vi "出账查询.vi"(9 "结束时间":timestamp format="%<%H:%M\n%y/%m/%d>T", 10 "起始时间":timestamp format="%<%H:%M\n%y/%m/%d>T", 11 "可选条件":bool) -> (1 "查询结果":string[][](table))   [LabVIEW 2010]
panel:
  out "error in (no error)":errorcluster caption="错误输入（无错误）"
  in  "表格控件":string[][](table)
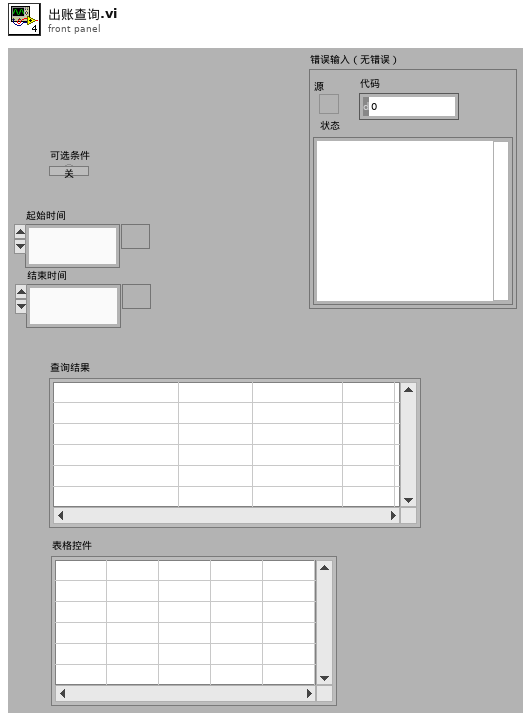
[diagram p1: front panel]
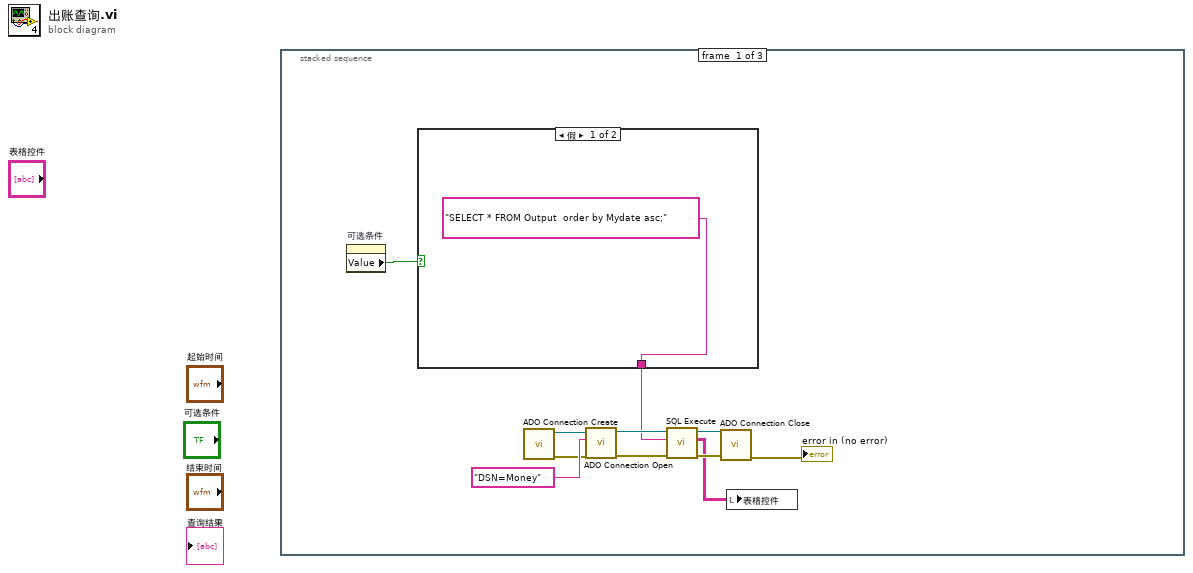
[diagram p0: block diagram]
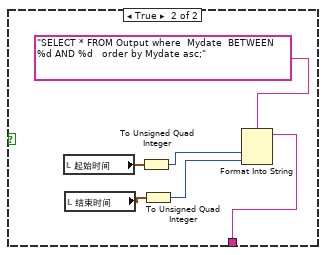
[diagram p2: hidden frame]
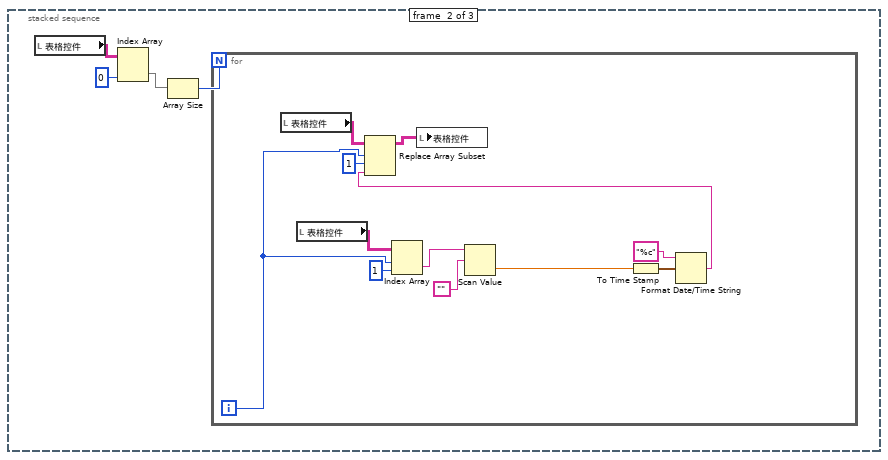
[diagram p3: hidden frame]
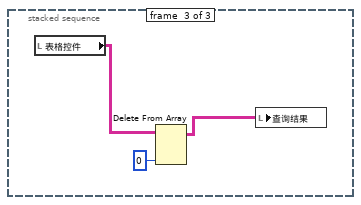
[diagram p4: hidden frame]
diagram:
  n1 = stacked-sequence {
    frame #0 {
      n2 = property on="可选条件" class="Bool (严格)"() -> ("Value"=w3:bool)  [unwired: 2 in, 2 out]
      n3 = case shown="假" w3 {
        tunnel: ["SELECT * FROM Output  order by Mydate asc;" w17] -> w2
        frame False {
        }
        frame True {
          n4 = local read "起始时间"() -> (w16:timestamp)
          n5 = local read "结束时间"() -> (w14:timestamp)
          n6 = To Unsigned Quad Integer(1:w16) -> (0:w15:u64)
          n7 = To Unsigned Quad Integer(1:w14) -> (0:w13:u64)
          n8 = Format Into String(format string="SELECT * FROM Output where  Mydate  BETWEEN %d AND %d   order by Mydate asc;", w15, w13) -> (resulting string=w17:string)  [unwired: 2 in, 1 out]
        }
      }
      n9 = call "ADO Connection Create.vi"() -> ("error out"=w5:errorcluster, "ADODB._Connection Out"=w6:refnum<k7>)  [unwired: 10 in]
      n10 = call "ADO Connection Open.vi"("error in (no error)"=w5, "ConnectionString"="DSN=Money", "ADODB._Connection In"=w6) -> ("error out"=w9:errorcluster, "ADODB._Connection Out"=w8:refnum<k7>)  [unwired: 7 in]
      n11 = call "SQL Execute.vi"("error in (no error)"=w9, "Command Text"=w2, "ADODB._Connection In"=w8) -> ("error out"=w11:errorcluster, "Data"=w1:string[][], "ADODB._Connection Out"=w10:refnum<k7>)  [unwired: 5 in, 1 out]
      n12 = call "ADO Connection Close.vi"("error in (no error)"=w11, "ADODB._Connection In"=w10) -> ("error out"=→"error in (no error)":errorcluster)  [unwired: 8 in, 1 out]
      n13 = local write "表格控件"(w1) -> ()
    }
    frame #1 {
      n14 = local read "表格控件"() -> (w20:string[][])
      n15 = Index Array(array=w20, index (col)=0 ("禁用的索引 (列)")) -> (element=w21:string[])  [unwired: 1 in]
      n16 = Array Size(array=w21) -> (size(s)=w19:i32)
      n17 = for {
        N: w19 -> [_]
        i -> [w23]
        n18 = local read "表格控件"() -> (w29:string[][])
        n19 = local read "表格控件"() -> (w27:string[][])
        n20 = Index Array(array=w27, index (row)=w23, index (col)=1 ("禁用的索引 (列)")) -> (element=w24:string)
        n21 = Scan Value(string=w24, format string="") -> (value=w32:dbl)  [unwired: 1 in, 1 out]
        n22 = To Time Stamp(1:w32) -> (0:w31:timestamp)
        n23 = Format Date/Time String(time format string (%c)="%c" ("时间格式字符串(%c)"), seconds (now)=w31) -> (date/time string=w25:string)  [unwired: 1 in]
        n24 = Replace Array Subset(array=w29, new element=w25, index (row)=w23, index (col)=1 ("禁用的索引 (列)")) -> (w28:string[][])
        n25 = local write "表格控件"(w28) -> ()
      }
    }
    frame #2 {
      n26 = local read "表格控件"() -> (w37:string[][])
      n27 = Delete From Array(array=w37, index (col)=0 ("禁用的索引 (列)")) -> (array with subset deleted=w36:string[][])  [unwired: 2 in, 1 out]
      n28 = local write "查询结果"(w36) -> ()
    }
  }
